vi "BMU诊断标定.vi"(5 "timeout":u32, 6 "Socket":dbl, 7 "通用配置?":bool, 8 "CAN端口":u16(ring), 9 "设备索引号":u16(ring), 10 "CAN卡类型":u32(ring)=21, 11 "从板号":u8=1) -> (3 "成功?":bool)   [LabVIEW 2013] (continued)
                    frame "从板信息" {
                    }
                    frame "电压个数" {
                    }
                    frame "通道电压节数" {
                    }
                    frame "保险位置" {
                    }
                    frame "温度个数" {
                    }
                    frame "风机关闭温差", "风机关闭温度", "风机开启温差", "风机开启温度", "加热关闭温差", "加热关闭温度", "加热开启温度", "加热控制参数" {
                    }
                    frame "SOC过低", "电压不均衡", "电压过低", "电压过高", "温度不均衡", "温度过低", "温度过高", "一级故障阀值" {
                    }
                    frame "SOC过低(2)", "电压不均衡(2)", "电压过低(2)", "电压过高(2)", "二级故障阀值", "温度不均衡(2)", "温度过低(2)", "温度过高(2)" {
                    }
                    frame "SOC过低(3)", "电压不均衡(3)", "电压过低(3)", "电压过高(3)", "三级故障阀值", "温度不均衡(3)", "温度过低(3)", "温度过高(3)" {
                    }
                    frame "快换参数" {
                    }
                    frame "均衡参数" {
                    }
                    frame "充电结束电压" {
                    }
                    frame "均衡阀值" {
                    }
                    frame "电池包信息1" {
                    }
                    frame "电池包序号" {
                    }
                    frame "充放电安时" {
                    }
                    frame "充电次数时间" {
                    }
                    frame "SOC" {
                    }
                    frame "车牌号" {
                    }
                    frame "充电参数" {
                    }
                  }
                  n3542 = local read "从板号"() -> (w4999:u8)
                }
              }
              n3543 = Build Array(w4914) -> (w4913:i32[])
              n3544 = local write "命令"(w4916) -> ()
              n3545 = Array Size(array=w4911) -> (size(s)=w4910:i32)
              n3546 = for {
                tunnel: w4911 -> [w5075] mode=indexing
                tunnel: w4916 -> [w5074]
                tunnel: w4915 -> [w5073]
                tunnel: w4913 -> [w5072]
                tunnel: w4912 -> [w5071] mode=indexing
                tunnel: w4910 -> [w5070]
                tunnel: w4909 -> [w5068]
                tunnel: [w5067] -> w4908
                i -> [w5069]
                n3547 = while {
                  tunnel: w5075 -> [w5084]
                  tunnel: w5074 -> [w5083]
                  tunnel: w5073 -> [w5082]
                  tunnel: w5072 -> [w5081]
                  tunnel: w5071 -> [w5080]
                  tunnel: w5070 -> [w5079]
                  tunnel: w5069 -> [w5078]
                  tunnel: w5068 -> [w5077]
                  tunnel: [w5076] -> w5067
                  stop <- w5076 stop-if-true
                  n3548 = stacked-sequence {
                    seq-local: [_ _ _ _ w5232 _ _] -> [_ _ _ _ _ w5241 _]
                    tunnel: w5084 -> [_ _ _ w5220 _ _ _]
                    tunnel: w5083 -> [_ _ _ w5219 _ _ _]
                    tunnel: w5082 -> [_ _ _ w5218 _ _ _]
                    tunnel: w5081 -> [_ _ _ w5217 _ _ _]
                    tunnel: [_ _ _ _ w5233 _ _] -> w5076
                    tunnel: w5080 -> [w5086 _ _ _ _ w5242 _]
                    tunnel: w5079 -> [_ _ _ _ _ _ w5252]
                    tunnel: w5078 -> [_ _ _ _ _ _ w5251]
                    tunnel: w5077 -> [w5085 _ _ _ _ _ _]
                    frame #0 {
                      n3549 = case shown="\"主板\", 默认" w5085 {
                        tunnel: w5086 -> [w5087 w5178]
                        frame "主板", Default {
                          n3550 = case shown="\"电压个数\"" w5087 {
                            frame "假", Default {
                            }
                            frame "产品编号" {
                              n3551 = control-ref of="产品编号"() -> (w5089:refnum<vi>)
                              n3552 = property class="Str"(reference=w5089, "Value"="") -> ()  [unwired: 1 in, 2 out]
                            }
                            frame "电压个数" {
                              n3553 = local read "从板个数"() -> (w5090:dbl)
                              n3554 = control-ref of="项目信息"() -> (w5094:refnum<vi>)
                              n3555 = for {
                                N: w5090 -> [_]
                                tunnel: [""] -> w5093 mode=indexing
                              }
                              n3556 = call "表格数据输入-8.6.vi"("行数"=u32 0, "列数"=u32 1, "字符串数组"=w5093, "表格引用"=w5094) -> ()  [unwired: 8 in]
                            }
                            frame "通道电压数" {
                              n3557 = control-ref of="项目信息"() -> (w5100:refnum<vi>)
                              n3558 = for {
                                N: 20 -> [_]
                                tunnel: [""] -> w5099 mode=indexing
                              }
                              n3559 = local read "从板个数"() -> (w5101:dbl)
                              n3560 = Increment(x=w5101) -> (x+1=w5097:dbl)
                              n3561 = call "表格数据输入-8.6.vi"("行数"=w5097, "列数"=u32 1, "字符串数组"=w5099, "表格引用"=w5100) -> ()  [unwired: 8 in]
                            }
                            frame "电压起始值" {
                              n3562 = local read "从板个数"() -> (w5105:dbl)
                              n3563 = Increment(x=w5105) -> (x+1=w5104:dbl)
                              n3564 = control-ref of="项目信息"() -> (w5111:refnum<vi>)
                              n3565 = for {
                                N: w5104 -> [_]
                                tunnel: [""] -> w5110 mode=indexing
                              }
                              n3566 = Multiply(x=u8 1, y=w5105) -> (x*y=w5107:dbl)
                              n3567 = Add(x=w5107, y=u8 21) -> (x+y=w5103:dbl)
                              n3568 = call "表格数据输入-8.6.vi"("行数"=w5103, "列数"=u32 1, "字符串数组"=w5110, "表格引用"=w5111) -> ()  [unwired: 8 in]
                            }
                            frame "温度个数" {
                              n3569 = local read "从板个数"() -> (w5115:dbl)
                              n3570 = Increment(x=w5115) -> (x+1=w5114:dbl)
                              n3571 = control-ref of="项目信息"() -> (w5121:refnum<vi>)
                              n3572 = for {
                                N: w5114 -> [_]
                                tunnel: [""] -> w5120 mode=indexing
                              }
                              n3573 = Multiply(x=u8 2, y=w5115) -> (x*y=w5117:dbl)
                              n3574 = Add(x=w5117, y=u8 22) -> (x+y=w5113:dbl)
                              n3575 = call "表格数据输入-8.6.vi"("行数"=w5113, "列数"=u32 1, "字符串数组"=w5120, "表格引用"=w5121) -> ()  [unwired: 8 in]
                            }
                            frame "温度起始值" {
                              n3576 = local read "从板个数"() -> (w5125:dbl)
                              n3577 = Increment(x=w5125) -> (x+1=w5124:dbl)
                              n3578 = control-ref of="项目信息"() -> (w5131:refnum<vi>)
                              n3579 = for {
                                N: w5124 -> [_]
                                tunnel: [""] -> w5130 mode=indexing
                              }
                              n3580 = Multiply(x=u8 3, y=w5125) -> (x*y=w5127:dbl)
                              n3581 = Add(x=w5127, y=u8 23) -> (x+y=w5123:dbl)
                              n3582 = call "表格数据输入-8.6.vi"("行数"=w5123, "列数"=u32 1, "字符串数组"=w5130, "表格引用"=w5131) -> ()  [unwired: 8 in]
                            }
                            frame "保险位置" {
                              n3583 = local read "从板个数"() -> (w5135:dbl)
                              n3584 = control-ref of="项目信息"() -> (w5141:refnum<vi>)
                              n3585 = for {
                                N: 10 -> [_]
                                tunnel: [""] -> w5140 mode=indexing
                              }
                              n3586 = Multiply(x=u8 4, y=w5135) -> (x*y=w5137:dbl)
                              n3587 = Add(x=w5137, y=u8 24) -> (x+y=w5134:dbl)
                              n3588 = call "表格数据输入-8.6.vi"("行数"=w5134, "列数"=u32 1, "字符串数组"=w5140, "表格引用"=w5141) -> ()  [unwired: 8 in]
                            }
                            frame "电池额定实际容量" {
                              w5143 = 0.0 ("值")
                              n3589 = control-ref of="电池实际容量(A)"() -> (w5144:refnum<vi>)
                              n3590 = control-ref of="电池额定容量(A)"() -> (w5145:refnum<vi>)
                              n3591 = property class="DigNum (严格)"(reference=w5144, "Value"=w5143) -> ()  [unwired: 1 in, 2 out]
                              n3592 = property class="DigNum (严格)"(reference=w5145, "Value"=w5143) -> ()  [unwired: 1 in, 2 out]
                            }
                            frame "SOC" {
                              n3593 = control-ref of="SOC(%)"() -> (w5146:refnum<vi>)
                              n3594 = property class="DigNum (严格)"(reference=w5146, "Value"=0.0 ("值")) -> ()  [unwired: 1 in, 2 out]
                            }
                            frame "配置文件版本" {
                              n3595 = control-ref of="配置文件版本"() -> (w5148:refnum<vi>)
                              n3596 = property class="Str"(reference=w5148, "Value"="" ("值")) -> ()  [unwired: 1 in, 2 out]
                            }
                            frame "参数修改记录" {
                              n3597 = control-ref of="使用者"() -> (w5151:refnum<vi>)
                              n3598 = control-ref of="系统时钟"() -> (w5152:refnum<vi>)
                              n3599 = property class="DigNum (严格)"(reference=w5151, "Value"=0.0 ("值")) -> ()  [unwired: 1 in, 2 out]
                              n3600 = property class="Str"(reference=w5152, "Value"="" ("值")) -> ()  [unwired: 1 in, 2 out]
                            }
                            frame "校正时钟" {
                              n3601 = control-ref of="系统时钟"() -> (w5154:refnum<vi>)
                              n3602 = property class="Str"(reference=w5154, "Value"="" ("值")) -> ()  [unwired: 1 in, 2 out]
                            }
                            frame "车牌号" {
                              n3603 = control-ref of="车架(牌)号"() -> (w5156:refnum<vi>)
                              n3604 = property class="Str"(reference=w5156, "Value"="" ("值")) -> ()  [unwired: 1 in, 2 out]
                            }
                            frame "SOH" {
                              n3605 = control-ref of="SOH(%)"() -> (w5159:refnum<vi>)
                              n3606 = property class="DigNum (严格)"(reference=w5159, "Value"=0.0 ("值")) -> ()  [unwired: 1 in, 2 out]
                            }
                            frame "一级故障阀值" {
                              n3607 = local write "一级故障"(T10 {"总电压过高"=0.0, "整组电压不均衡"=0.0, "SOC过高"=0.0, "单体电压过高"=0.0, "总电压过低"=0.0, "温度过高"=0.0, "温度过低"=0.0, "单组电压不均衡"=0.0, "整组温度不均衡"=0.0, "单组温度不均衡"=0.0, "单体电压过低"=0.0, "充电电流过高"=0.0, "放电电流过高"=0.0, "SOC过低"=0.0, "内阻过大"=0.0, "极柱温度过高"=0.0, "SOH过低"=0.0} ("一级故障")) -> ()
                            }
                            frame "二级故障阀值" {
                              n3608 = local write "一级故障 2"(T10 {"总电压过高"=0.0, "整组电压不均衡"=0.0, "SOC过高"=0.0, "单体电压过高"=0.0, "总电压过低"=0.0, "温度过高"=0.0, "温度过低"=0.0, "单组电压不均衡"=0.0, "整组温度不均衡"=0.0, "单组温度不均衡"=0.0, "单体电压过低"=0.0, "充电电流过高"=0.0, "放电电流过高"=0.0, "SOC过低"=0.0, "内阻过大"=0.0, "极柱温度过高"=0.0, "SOH过低"=0.0} ("一级故障")) -> ()
                            }
                            frame "三级故障阀值" {
                              n3609 = local write "一级故障 3"(T10 {"总电压过高"=0.0, "整组电压不均衡"=0.0, "SOC过高"=0.0, "单体电压过高"=0.0, "总电压过低"=0.0, "温度过高"=0.0, "温度过低"=0.0, "单组电压不均衡"=0.0, "整组温度不均衡"=0.0, "单组温度不均衡"=0.0, "单体电压过低"=0.0, "充电电流过高"=0.0, "放电电流过高"=0.0, "SOC过低"=0.0, "内阻过大"=0.0, "极柱温度过高"=0.0, "SOH过低"=0.0} ("一级故障")) -> ()
                            }
                            frame "加热控制参数" {
                              n3610 = local write "加热控制参数"(T11 {"风机开启温度"=0.0, "风机关闭温度"=0.0, "加热开启温度"=0.0, "加热关闭温度"=0.0, "风机开启温差"=0.0, "风机关闭温差"=0.0, "加热关闭温差"=0.0} ("加热控制参数")) -> ()
                            }
                            frame "充电控制参数" {
                              n3611 = local write "一级故障 5"(T12 {"最大允许单体电压"=0.0, "最大允许总电压"=0.0, "最小允许单体电压"=0.0, "最大允许充电电流"=0.0, "最小允许充电电流"=0.0, "最大允许充电温度"=0.0, "最小允许充电温度"=0.0, "电流步长"=0.0} ("一级故障 5")) -> ()
                            }
                            frame "电池信息1" {
                              w5165 = ""
                              w5166 = 0.0 ("电池串联")
                              n3612 = local read "电池信息"() -> (w5168:T13)
                              n3613 = Bundle By Name(cluster=w5168, "电池串联"=w5166, "电池并联"=w5166, "电池包额定容量"=w5166, "电池包额定能量(kWh)"=w5166, "电池包额定总电压"=w5166, "实际容量"=w5166, "电池厂家"=w5165, "电池类型"=w5165, "电池生产日期"=w5165) -> (w5167:T13)
                              n3614 = local write "电池信息"(w5167) -> ()
                            }
                            frame "电池包组号" {
                              n3615 = local read "电池信息"() -> (w5171:T13)
                              n3616 = Bundle By Name(cluster=w5171, "电池包组号"="") -> (w5170:T13)
                              n3617 = local write "电池信息"(w5170) -> ()
                            }
                            frame "充放电安时" {
                              w5172 = 0.0 ("累计充电总安时")
                              n3618 = local read "电池信息"() -> (w5174:T13)
                              n3619 = Bundle By Name(cluster=w5174, "累计充电总安时"=w5172, "累计放电总安时"=w5172) -> (w5173:T13)
                              n3620 = local write "电池信息"(w5173) -> ()
                            }
                            frame "电池充放电次数" {
                              w5175 = 0.0 ("累计充电总安时")
                              n3621 = local read "电池信息"() -> (w5177:T13)
                              n3622 = Bundle By Name(cluster=w5177, "电池充满次数"=w5175, "电池放空次数"=w5175, "电池充电次数"=w5175) -> (w5176:T13)
                              n3623 = local write "电池信息"(w5176) -> ()
                            }
                          }
                        }
                        frame "从板" {
                          n3624 = case shown="\"加热控制参数\"" w5178 {
                            frame "假", Default {
                            }
                            frame "电压起始值" {
                              n3625 = control-ref of="项目信息 2"() -> (w5180:refnum<vi>)
                              n3626 = for {
                                N: 1 -> [_]
                                tunnel: [""] -> w5183 mode=indexing
                              }
                              n3627 = call "表格数据输入-8.6.vi"("行数"=u32 0, "列数"=u32 1, "字符串数组"=w5183, "表格引用"=w5180) -> ()  [unwired: 8 in]
                            }
                            frame "通道电压节数" {
                              n3628 = control-ref of="项目信息 2"() -> (w5185:refnum<vi>)
                              n3629 = for {
                                N: 5 -> [_]
                                tunnel: [""] -> w5189 mode=indexing
                              }
                              n3630 = call "表格数据输入-8.6.vi"("行数"=u32 22, "列数"=u32 1, "字符串数组"=w5189, "表格引用"=w5185) -> ()  [unwired: 8 in]
                            }
                            frame "保险位置" {
                              n3631 = control-ref of="项目信息 2"() -> (w5191:refnum<vi>)
                              n3632 = for {
                                N: 20 -> [_]
                                tunnel: [""] -> w5195 mode=indexing
                              }
                              n3633 = call "表格数据输入-8.6.vi"("行数"=u32 2, "列数"=u32 1, "字符串数组"=w5195, "表格引用"=w5191) -> ()  [unwired: 8 in]
                            }
                            frame "温度起始值" {
                              n3634 = control-ref of="项目信息 2"() -> (w5197:refnum<vi>)
                              n3635 = for {
                                N: 1 -> [_]
                                tunnel: [""] -> w5201 mode=indexing
                              }
                              n3636 = call "表格数据输入-8.6.vi"("行数"=u32 1, "列数"=u32 1, "字符串数组"=w5201, "表格引用"=w5197) -> ()  [unwired: 8 in]
                            }
                            frame "加热控制参数" {
                              n3637 = local write "加热控制参数"(T11 {"风机开启温度"=0.0, "风机关闭温度"=0.0, "加热开启温度"=0.0, "加热关闭温度"=0.0, "风机开启温差"=0.0, "风机关闭温差"=0.0, "加热关闭温差"=0.0} ("加热控制参数")) -> ()
                            }
                            frame "一级故障阀值" {
                              n3638 = local write "一级故障 6"(T15 {"电压过高"=0.0, "电压过低"=0.0, "温度过高"=0.0, "温度过低"=0.0, "电压不均衡(V)"=0.0, "温度不均衡"=0.0, "SOC过低"=0.0} ("一级故障 6")) -> ()
                            }
                            frame "二级故障阀值" {
                              n3639 = local write "一级故障 7"(T15 {"电压过高"=0.0, "电压过低"=0.0, "温度过高"=0.0, "温度过低"=0.0, "电压不均衡(V)"=0.0, "温度不均衡"=0.0, "SOC过低"=0.0} ("一级故障 7")) -> ()
                            }
                            frame "三级故障阀值" {
                              n3640 = local write "一级故障 8"(T15 {"电压过高"=0.0, "电压过低"=0.0, "温度过高"=0.0, "温度过低"=0.0, "电压不均衡(V)"=0.0, "温度不均衡"=0.0, "SOC过低"=0.0} ("一级故障 7")) -> ()
                            }
                            frame "均衡参数" {
                              n3641 = local write "均衡参数"(T17 {"充电结束电压(90%)"=0.0, "充电结束电压(91%)"=0.0, "充电结束电压(92%)"=0.0, "充电结束电压(93%)"=0.0, "充电结束电压(94%)"=0.0, "均衡计算-电压高阀值1级"=0.0, "均衡计算-电压高阀值2级"=0.0, "均衡计算-电压低阀值1级"=0.0, "均衡计算-电压低阀值2级"=0.0, "均衡计算-最低电压阀值"=0.0, "均衡停止-最低电压阀值"=0.0, "均衡计算-电压极差阀值"=0.0, "充电结束电压(95%)"=0.0, "充电结束电压(96%)"=0.0, "充电结束电压(97%)"=0.0, "充电结束电压(98%)"=0.0, "充电结束电压(99%)"=0.0, "充电结束电压(100%)"=0.0} ("均衡参数")) -> ()
                            }
                            frame "均衡阀值" {
                              w5208 = sgl 0.0 ("均衡计算-电压高阀值1级")
                              n3642 = local read "均衡参数"() -> (w5209:T17)
                              n3643 = Bundle By Name(cluster=w5209, "均衡计算-电压高阀值1级"=w5208, "均衡计算-电压高阀值2级"=w5208, "均衡计算-电压低阀值1级"=w5208, "均衡计算-电压低阀值2级"=w5208, "均衡计算-最低电压阀值"=w5208, "均衡停止-最低电压阀值"=w5208, "均衡计算-电压极差阀值"=w5208) -> (w5210:T17)
                              n3644 = local write "均衡参数"(w5210) -> ()
                            }
                            frame "充电结束电压" {
                              w5211 = sgl 0.0 ("均衡计算-电压高阀值1级")
                              n3645 = local read "均衡参数"() -> (w5212:T17)
                              n3646 = Bundle By Name(cluster=w5212, "充电结束电压(90%)"=w5211, "充电结束电压(91%)"=w5211, "充电结束电压(92%)"=w5211, "充电结束电压(93%)"=w5211, "充电结束电压(94%)"=w5211, "充电结束电压(95%)"=w5211, "充电结束电压(96%)"=w5211, "充电结束电压(97%)"=w5211, "充电结束电压(98%)"=w5211, "充电结束电压(99%)"=w5211, "充电结束电压(100%)"=w5211) -> (w5213:T17)
                              n3647 = local write "均衡参数"(w5213) -> ()
                            }
                          }
                        }
                      }
                    }
                    frame #1 {
                      w5214 = FALSE ("流控帧")
                      w5215 = TRUE ("流控帧 2")
                      n3648 = global write "EV05全局变量1.vi" "写入超时"(w5214) -> ()
                      n3649 = global write "EV05全局变量1.vi" "流控帧"(w5214) -> ()
                      n3650 = local write "写?"(w5214) -> ()
                      n3651 = call <vilib>:"Set Busy.vi"("disable click? (T)"=w5214) -> ()  [unwired: 3 in, 8 out]
                      n3652 = local write "消除"(w5215) -> ()
                      n3653 = local write "控制1"(w5215) -> ()
                      n3654 = global write "EV05全局变量1.vi" "流控帧 2"(w5215) -> ()
                    }
                    frame #2 {
                      n3655 = Wait Until Next ms Multiple(millisecond multiple=u32 150 ("毫秒倍数")) -> ()  [unwired: 1 out]
                    }
                    frame #3 {
                      n3656 = local read "设备索引号"() -> (w5222:u16)
                      n3657 = local read "CAN卡类型"() -> (w5223:u32)
                      n3658 = local read "CAN端口"() -> (w5221:u16)
                      n3659 = stacked-sequence {
                        tunnel: w5223 -> [_ w5231]
                        tunnel: w5222 -> [_ w5230]
                        tunnel: w5221 -> [_ w5229]
                        tunnel: w5220 -> [_ w5228]
                        tunnel: w5219 -> [_ w5227]
                        tunnel: w5218 -> [_ w5226]
                        tunnel: w5217 -> [_ w5225]
                        frame #0 {
                        }
                        frame #1 {
                          n3660 = call "多帧发送机制(EV05).vi"("can卡类型"=w5231, "设备索引号"=w5230, "CAN端口"=w5229, "命令"=w5227, "板号"=w5226, "命令序号"=w5228, "输入数据"=w5225) -> ("错误输出"=w5224:errorcluster)  [unwired: 2 in, 10 out]
                          n3661 = call <vilib>:"Clear Errors.vi"("error in (no error)"=w5224) -> ()  [unwired: 6 in, 1 out]
                        }
                      }
                      "命令序号" <- w5220
                    }
                    frame #4 {
                      n3662 = while {
                        tunnel: [w5236] -> w5233
                        tunnel: [w5235] -> w5232
                        i -> [w5239]
                        stop <- w5236 stop-if-true
                        n3663 = local read "强制终止读写标记"() -> (w5234:bool)
                        n3664 = global read "EV05全局变量1.vi" "写入超时"() -> (w5235:bool)
                        n3665 = Greater Or Equal?(x=w5239, y=30) -> (x >= y?=w5237:bool)
                        n3666 = Compound Arithmetic op=OR(w5234, w5235, w5237) -> (w5236:bool)
                        n3667 = Wait Until Next ms Multiple(millisecond multiple=u32 100 ("毫秒倍数")) -> ()  [unwired: 1 out]
                      }
                    }
                    frame #5 {
                      n3668 = call <vilib>:"Unset Busy.vi"() -> ()  [unwired: 11 in, 1 out]
                      n3669 = case shown="假" w5241 {
                        tunnel: w5242 -> [w5245 _]
                        frame False {
                          n3670 = control-ref of="结果"() -> (w5244:refnum<vi>)
                          n3671 = Concatenate Strings(w5245, "     读取失败" ("字符串")) -> (w5247:string)
                          n3672 = Build Array(w5247) -> (w5243:string[])
                          n3673 = call "表格编辑.vi"("新元素/子数组"=w5243, "活动单元格:单元格背景色"=u32 16740749, "MCListbox引用句柄"=w5244) -> ()  [unwired: 9 out]
                        }
                        frame True {
                        }
                      }
                    }
                    frame #6 {
                      n3674 = Increment(x=w5251) -> (x+1=w5250:i32)
                      n3675 = Equal?(x=w5252, y=w5250) -> (x = y?=w5249:bool)
                      n3676 = case shown="真" w5249 {
                        frame False {
                        }
                        frame True {
                          n3677 = control-ref of="结果"() -> (w5254:refnum<vi>)
                          n3678 = Concatenate Strings("读取完成" ("字符串")) -> (w5256:string)
                          n3679 = Build Array(w5256) -> (w5253:string[])
                          n3680 = call "表格编辑.vi"("新元素/子数组"=w5253, "活动单元格:单元格背景色"=u32 21937, "MCListbox引用句柄"=w5254) -> ()  [unwired: 9 out]
                        }
                      }
                    }
                  }
                }
              }
            }
          }
          n3681 = stacked-sequence {
            tunnel: w4906 -> [_]
            frame #0 {
              n3682 = call <vilib>:"Unset Busy.vi"() -> ()  [unwired: 11 in, 1 out]
              n3683 = local write "强制终止读写标记"(FALSE ("强制停止")) -> ()
            }
          }
        }
        frame "全部读取" {
          n3684 = stacked-sequence {
            seq-local: [w5262 _ _] -> [_ _ w5817]
            seq-local: [w5261 _ _] -> [_ _ w5816]
            tunnel: [_ w5453 _] -> w5259
            frame #0 {
              n3685 = local read "主从选择"() -> (w5262:enum32{"主板", "从板"})
              n3686 = local read "路径"() -> (w5263:path)
              n3687 = Empty String/Path?(string/path=w5263) -> (empty?=w5261:bool)
              n3688 = disable-structure shown="禁用" {
                disable-tunnel: w5263 -> [w5266 _]
                disable-tunnel: w5261 -> [w5265 _]
                disable-tunnel: w5262 -> [w5264 _]
                frame Disabled {
                  n3689 = case shown="假" w5265 {
                    tunnel: w5266 -> [w5270 _]
                    tunnel: w5264 -> [w5269 _]
                    frame False {
                      n3690 = control-ref of="结果"() -> (w5267:refnum<vi>)
                      n3691 = call-poly <vilib>:"Read From Spreadsheet File.vi"("file path (dialog if empty)"=w5270) -> ("all rows"=w5268:string[][])  [unwired: 3 in, 7 out]
                      n3692 = case shown="\"主板\", 默认" w5269 {
                        tunnel: w5268 -> [w5272 w5367]
                        tunnel: w5267 -> [w5271 w5366]
                        frame "主板", Default {
                          n3693 = stacked-sequence {
                            tunnel: w5272 -> [w5281 w5305 w5362]
                            tunnel: w5271 -> [w5278 _ w5333]
                            frame #0 {
                              n3694 = Index Array(array=w5281, index (col)=3 ("禁用的索引 (列)")) -> (element=w5295:string[])  [unwired: 1 in]
                              n3695 = Index Array(array=w5281, index (col)=1 ("禁用的索引 (列)")) -> (element=w5301:string[])  [unwired: 1 in]
                              n3696 = Delete From Array(array=w5295, length=4 ("长度"), index=0 ("索引")) -> (deleted portion=w5292:string[], array with subset deleted=w5286:string[])
                              n3697 = Delete From Array(array=w5301, length=1 ("长度"), index=0 ("索引")) -> (deleted portion=w5298:string[], array with subset deleted=w5275:string[])
                              n3698 = Build Array("正在读取主板配置文件...") -> (w5279:string[])
                              n3699 = Index Array(array=w5286) -> (element #1=w5285:string, element #2=w5284:string, element #3=w5283:string, element #4=w5282:string)  [unwired: 4 in]
                              n3700 = for {
                                tunnel: w5292 -> [w5304] mode=indexing
                                tunnel: [w5303] -> w5291 mode=indexing
                                n3701 = Fract/Exp String To Number(string=w5304) -> (number=w5303:dbl)  [unwired: 4 out]
                              }
                              n3702 = Index Array(array=w5298) -> (element=w5297:string)  [unwired: 1 in]
                              n3703 = global write "读配置文件全局.vi" "表格输入"(w5275) -> ()
                              n3704 = call "表格编辑.vi"("新元素/子数组"=w5279, "活动单元格:单元格背景色"=u32 6618880, "MCListbox引用句柄"=w5278) -> ()  [unwired: 9 out]
                              n3705 = Decimal String To Number(string=w5297) -> (number=w5276:i32)  [unwired: 1 in, 2 out]
                              n3706 = global read "读配置文件全局.vi" "项目信息"() -> (w5274:T27)
                              n3707 = Index Array(array=w5291) -> (element #1=w5290:dbl, element #2=w5289:dbl, element #3=w5288:dbl, element #4=w5287:dbl)  [unwired: 4 in]
                              n3708 = global write "读配置文件全局.vi" "从板个数"(w5276) -> ()
                              n3709 = Bundle(cluster=w5274, "电池额定容量"=w5290, "电池实际容量"=w5289, "车牌号"=w5285, "配置文件版本"=w5284, "SOH"=w5287, "SOC"=w5288, "产品编号"=w5283, "系统时钟"=w5282) -> (w5273:T27)  [unwired: 1 out]
                              n3710 = global write "读配置文件全局.vi" "项目信息"(w5273) -> ()
                            }
                            frame #1 {
                              n3711 = Index Array(array=w5305, index (col)=3 ("禁用的索引 (列)")) -> (element=w5323:string[])  [unwired: 1 in]
                              n3712 = Index Array(array=w5305, index (col)=5 ("禁用的索引 (列)")) -> (element=w5317:string[])  [unwired: 1 in]
                              n3713 = for {
                                tunnel: w5317 -> [w5330] mode=indexing
                                tunnel: [w5329] -> w5316 mode=indexing
                                n3714 = Fract/Exp String To Number(string=w5330) -> (number=w5329:dbl)  [unwired: 4 out]
                              }
                              n3715 = Delete From Array(array=w5323, length=17 ("长度"), index=8 ("索引")) -> (deleted portion=w5321:string[])  [unwired: 1 out]
                              n3716 = for {
                                tunnel: w5321 -> [w5332] mode=indexing
                                tunnel: [w5331] -> w5319 mode=indexing
                                n3717 = Fract/Exp String To Number(string=w5332) -> (number=w5331:dbl)  [unwired: 4 out]
                              }
                              n3718 = global write "读配置文件全局.vi" "二级故障"(w5316) -> ()
                              n3719 = global write "读配置文件全局.vi" "一级故障"(w5319) -> ()
                              n3720 = Index Array(array=w5305, index (col)=7 ("禁用的索引 (列)")) -> (element=w5314:string[])  [unwired: 1 in]
                              n3721 = Index Array(array=w5305, index (col)=9 ("禁用的索引 (列)")) -> (element=w5311:string[])  [unwired: 1 in]
                              n3722 = for {
                                tunnel: w5314 -> [w5328] mode=indexing
                                tunnel: [w5327] -> w5313 mode=indexing
                                n3723 = Fract/Exp String To Number(string=w5328) -> (number=w5327:dbl)  [unwired: 4 out]
                              }
                              n3724 = for {
                                tunnel: w5311 -> [w5326] mode=indexing
                                tunnel: [w5325] -> w5310 mode=indexing
                                n3725 = Fract/Exp String To Number(string=w5326) -> (number=w5325:dbl)  [unwired: 4 out]
                              }
                              n3726 = Delete From Array(array=w5310, length=6 ("长度"), index=0 ("索引")) -> (deleted portion=w5307:dbl[], array with subset deleted=w5306:dbl[])
                              n3727 = global write "读配置文件全局.vi" "三级故障"(w5313) -> ()
                              n3728 = global write "读配置文件全局.vi" "加热控制参数"(w5307) -> ()
                              n3729 = global write "读配置文件全局.vi" "充电控制参数"(w5306) -> ()
                            }
                            frame #2 {
                              n3730 = call <vilib>:"Unset Busy.vi"() -> ()  [unwired: 2 in, 10 out]
                              n3731 = Index Array(array=w5362, index (col)=11 ("禁用的索引 (列)")) -> (element=w5359:string[])  [unwired: 1 in]
                              n3732 = Delete From Array(array=w5359, length=6 ("长度"), index=0 ("索引")) -> (deleted portion=w5341:string[], array with subset deleted=w5340:string[])
                              n3733 = for {
                                tunnel: w5340 -> [w5365] mode=indexing
                                tunnel: [w5364] -> w5358 mode=indexing
                                n3734 = Fract/Exp String To Number(string=w5365) -> (number=w5364:dbl)  [unwired: 4 out]
                              }
                              n3735 = Index Array(array=w5341) -> (element #1=w5357:string, element #2=w5356:string, element #3=w5355:string, element #4=w5354:string, element #5=w5353:string, element #6=w5352:string)  [unwired: 6 in]
                              n3736 = Index Array(array=w5358) -> (element #1=w5351:dbl, element #2=w5350:dbl, element #3=w5349:dbl, element #4=w5348:dbl, element #5=w5347:dbl, element #6=w5346:dbl, element #7=w5345:dbl, element #8=w5344:dbl, element #9=w5343:dbl, element #10=w5342:dbl, element #11=w5337:dbl)  [unwired: 11 in]
                              n3737 = global read "读配置文件全局.vi" "电池信息"() -> (w5339:T28)
                              n3738 = Build Array("配置文件读取完成") -> (w5335:string[])
                              n3739 = Bundle(cluster=w5339, "电池串联"=w5351, "电池并联"=w5350, "累计放电总安时"=w5348, "电池包额定容量"=w5347, "电池包额定能量"=w5346, "电池包额定总电压"=w5345, "累计充电总安时"=w5349, "电池充满次数"=w5344, "电池放空次数"=w5343, "电池充电次数"=w5342, "电池生产日期"=w5357, "电池厂家"=w5356, "电池类型"=w5355, "电池包组号"=w5354, "电池包产权标识"=w5353, "电池应用车型"=w5352, "实际容量"=w5337) -> (w5338:T28)
                              n3740 = call "表格编辑.vi"("新元素/子数组"=w5335, "活动单元格:单元格背景色"=u32 6618880, "MCListbox引用句柄"=w5333) -> ()  [unwired: 9 out]
                              n3741 = global write "读配置文件全局.vi" "电池信息"(w5338) -> ()
                            }
                          }
                        }
                        frame "从板" {
                          n3742 = stacked-sequence {
                            tunnel: w5367 -> [w5375 w5403 w5447]
                            tunnel: w5366 -> [w5372 _ w5423]
                            frame #0 {
                              n3743 = Index Array(array=w5375, index (col)=1 ("禁用的索引 (列)")) -> (element=w5385:string[])  [unwired: 1 in]
                              n3744 = Index Array(array=w5375, index (col)=3 ("禁用的索引 (列)")) -> (element=w5379:string[])  [unwired: 1 in]
                              n3745 = Delete From Array(array=w5385, length=1 ("长度"), index=0 ("索引")) -> (deleted portion=w5382:string[], array with subset deleted=w5369:string[])
                              n3746 = Delete From Array(array=w5379, length=6 ("长度"), index=0 ("索引")) -> (deleted portion=w5376:string[])  [unwired: 1 out]
                              n3747 = for {
                                tunnel: w5376 -> [w5388] mode=indexing
                                tunnel: [w5387] -> w5368 mode=indexing
                                i -> [w5389]
                                n3748 = Fract/Exp String To Number(string=w5388, default (0 dbl)=w5389) -> (number=w5387:i32)  [unwired: 3 out]
                              }
                              n3749 = Index Array(array=w5382) -> (element=w5381:string)  [unwired: 1 in]
                              n3750 = global write "读配置文件全局2.vi" "表格"(w5369) -> ()
                              n3751 = Build Array("正在读取从板配置文件...") -> (w5373:string[])
                              n3752 = Decimal String To Number(string=w5381) -> (number=w5370:i32)  [unwired: 1 in, 2 out]
                              n3753 = call "表格编辑.vi"("新元素/子数组"=w5373, "活动单元格:单元格背景色"=u32 6618880, "MCListbox引用句柄"=w5372) -> ()  [unwired: 9 out]
                              n3754 = global write "读配置文件全局2.vi" "加热控制参数"(w5368) -> ()
                              n3755 = global write "读配置文件全局2.vi" "从板板号"(w5370) -> ()
                            }
                            frame #1 {
                              n3756 = Index Array(array=w5403, index (col)=3 ("禁用的索引 (列)")) -> (element=w5393:string[])  [unwired: 1 in]
                              n3757 = Array Subset(array=w5393, index=6 ("索引"), length=7 ("长度")) -> (w5400:string[])
                              n3758 = Array Subset(array=w5393, index=13 ("索引"), length=7 ("长度")) -> (w5399:string[])
                              n3759 = Array Subset(array=w5393, index=20 ("索引"), length=7 ("长度")) -> (w5394:string[])
                              n3760 = for {
                                tunnel: w5400 -> [w5410] mode=indexing
                                tunnel: [w5409] -> w5390 mode=indexing
                                n3761 = Fract/Exp String To Number(string=w5410) -> (number=w5409:dbl)  [unwired: 4 out]
                              }
                              n3762 = for {
                                tunnel: w5399 -> [w5408] mode=indexing
                                tunnel: [w5407] -> w5391 mode=indexing
                                n3763 = Fract/Exp String To Number(string=w5408) -> (number=w5407:dbl)  [unwired: 4 out]
                              }
                              n3764 = for {
                                tunnel: w5394 -> [w5406] mode=indexing
                                tunnel: [w5405] -> w5392 mode=indexing
                                n3765 = Fract/Exp String To Number(string=w5406) -> (number=w5405:dbl)  [unwired: 4 out]
                              }
                              n3766 = global write "读配置文件全局2.vi" "一级故障阀值"(w5390) -> ()
                              n3767 = global write "读配置文件全局2.vi" "二级故障阀值"(w5391) -> ()
                              n3768 = global write "读配置文件全局2.vi" "三级故障阀值"(w5392) -> ()
                            }
                            frame #2 {
                              n3769 = Index Array(array=w5447, index (col)=5 ("禁用的索引 (列)")) -> (element=w5445:string[])  [unwired: 1 in]
                              n3770 = Delete From Array(array=w5445, length=1 ("长度"), index=16 ("索引")) -> (deleted portion=w5441:string[], array with subset deleted=w5442:string[])
                              n3771 = for {
                                tunnel: w5442 -> [w5450] mode=indexing
                                tunnel: [w5449] -> w5446 mode=indexing
                                n3772 = Fract/Exp String To Number(string=w5450) -> (number=w5449:dbl)  [unwired: 4 out]
                              }
                              n3773 = Index Array(array=w5446) -> (element #1=w5440:dbl, element #2=w5439:dbl, element #3=w5438:dbl, element #4=w5437:dbl, element #5=w5436:dbl, element #6=w5435:dbl, element #7=w5434:dbl, element #8=w5433:dbl, element #9=w5432:dbl, element #10=w5431:dbl, element #11=w5430:dbl, element #12=w5421:dbl, element #13=w5429:dbl, element #14=w5428:dbl, element #15=w5427:dbl, element #16=w5426:dbl, element #17=w5419:dbl, element #18=w5418:dbl, element #19=w5417:dbl, element #20=w5416:dbl, element #21=w5415:dbl, element #22=w5414:dbl)  [unwired: 22 in]
                              n3774 = Build Array("配置文件读取完成") -> (w5424:string[])
                              n3775 = Index Array(array=w5441, index=22 ("索引")) -> (element=w5420:string)
                              n3776 = global read "读配置文件全局2.vi" "电池组信息"() -> (w5412:T29)
                              n3777 = call "表格编辑.vi"("新元素/子数组"=w5424, "活动单元格:单元格背景色"=u32 6618880, "MCListbox引用句柄"=w5423) -> ()  [unwired: 9 out]
                              n3778 = Bundle(cluster=w5412, "电池类型"=w5440, "电池厂家"=w5439, "电池地区"=w5438, "电池组序号"=w5437, "电池包串联数"=w5436, "电池包并联数"=w5435, "电池包安时数"=w5434, "电池包序号"=w5433, "充电次数"=w5432, "充满电时间"=w5431, "放空时间"=w5430, "车牌号"=w5420, "最大允许单体电压"=w5421, "最大允许总电压"=w5429, "最大允许温度"=w5428, "最小允许温度"=w5427, "最大允许充电电流"=w5426, "最小允许充电电流"=w5419, "最小允许单体电压"=w5418, "电流步长"=w5417, "SOC"=w5416, "充电总安时"=w5415, "放电总这时"=w5414) -> (w5411:T29)
                              n3779 = call <vilib>:"Unset Busy.vi"() -> ()  [unwired: 2 in, 10 out]
                              n3780 = global write "读配置文件全局2.vi" "电池组信息"(w5411) -> ()
                            }
                          }
                        }
                      }
                    }
                    frame True {
                    }
                  }
                }
                frame Enabled {
                }
              }
              n3781 = case shown="\"从板\"" w5262 {
                frame "主板", Default {
                  w5451 = FALSE
                  n3782 = global write "读配置文件全局.vi" "SOC判定"(w5451) -> ()
                  n3783 = global write "读配置文件全局.vi" "SOH判定"(w5451) -> ()
                  n3784 = global write "读配置文件全局.vi" "车牌号判定"(w5451) -> ()
                  n3785 = global write "读配置文件全局.vi" "电池信息1判定"(w5451) -> ()
                  n3786 = global write "读配置文件全局.vi" "保险位置判定"(w5451) -> ()
                  n3787 = global write "读配置文件全局.vi" "产品编号判定"(w5451) -> ()
                  n3788 = global write "读配置文件全局.vi" "充放电安时判定"(w5451) -> ()
                  n3789 = global write "读配置文件全局.vi" "从板个数判定"(w5451) -> ()
                  n3790 = global write "读配置文件全局.vi" "电池包组号判定"(w5451) -> ()
                  n3791 = global write "读配置文件全局.vi" "电压个数判定"(w5451) -> ()
                  n3792 = global write "读配置文件全局.vi" "电压起始值判定"(w5451) -> ()
                  n3793 = global write "读配置文件全局.vi" "二级故障判定"(w5451) -> ()
                  n3794 = global write "读配置文件全局.vi" "三级故障判定"(w5451) -> ()
                  n3795 = global write "读配置文件全局.vi" "通道电压数判定"(w5451) -> ()
                  n3796 = global write "读配置文件全局.vi" "温度个数判定"(w5451) -> ()
                  n3797 = global write "读配置文件全局.vi" "一级故障判定"(w5451) -> ()
                  n3798 = global write "读配置文件全局.vi" "温度起始值判定"(w5451) -> ()
                  n3799 = global write "读配置文件全局.vi" "充电控制参数判定"(w5451) -> ()
                  n3800 = global write "读配置文件全局.vi" "电池充放电次数判定"(w5451) -> ()
                  n3801 = global write "读配置文件全局.vi" "加热控制参数判定"(w5451) -> ()
                  n3802 = global write "读配置文件全局.vi" "配置文件版本判定"(w5451) -> ()
                  n3803 = global write "读配置文件全局.vi" "电池额定实际容量判定"(w5451) -> ()
                }
                frame "从板" {
                  w5452 = FALSE
                  n3804 = disable-structure shown="禁用" {
                    frame Disabled {
                      n3805 = global read "读配置文件全局2.vi" "充电次数时间判定"() -> ()  [unwired: 1 in]
                      n3806 = global read "读配置文件全局2.vi" "电池包信息1判定"() -> ()  [unwired: 1 in]
                      n3807 = global read "读配置文件全局2.vi" "电池包序号判定"() -> ()  [unwired: 1 in]
                      n3808 = global read "读配置文件全局2.vi" "充放电安时判定"() -> ()  [unwired: 1 in]
                      n3809 = global read "读配置文件全局2.vi" "车牌号判定"() -> ()  [unwired: 1 in]
                      n3810 = global read "读配置文件全局2.vi" "充电参数判定"() -> ()  [unwired: 1 in]
                      n3811 = global read "读配置文件全局2.vi" "保险位置判定"() -> ()  [unwired: 1 in]
                    }
                    frame Enabled {
                    }
                  }
                  n3812 = global write "读配置文件全局2.vi" "从板号判定"(w5452) -> ()
                  n3813 = global write "读配置文件全局2.vi" "通道电压判定"(w5452) -> ()
                  n3814 = global write "读配置文件全局2.vi" "保险位置判定"(w5452) -> ()
                  n3815 = global write "读配置文件全局2.vi" "二级故障判定"(w5452) -> ()
                  n3816 = global write "读配置文件全局2.vi" "三级故障判定"(w5452) -> ()
                  n3817 = global write "读配置文件全局2.vi" "一级故障判定"(w5452) -> ()
                  n3818 = global write "读配置文件全局2.vi" "电压起始值判定"(w5452) -> ()
                  n3819 = global write "读配置文件全局2.vi" "温度起始值判定"(w5452) -> ()
                }
              }
            }
            frame #1 {
              (unwired) "均衡参数"
              # "去掉加热控制信息 20140106"
              n3820 = local read "主从选择"() -> (w5456:enum32{"主板", "从板"})
              n3821 = case shown="\"主板\", 默认" w5456 {
                tunnel: [string[] ["项目信息", "一级故障阀值", "二级故障阀值", "三级故障阀值", "加热控制信息", "充电控制信息", "电池信息"] string[] ["从板信息", "一级故障阀值", "二级故障阀值", "三级故障阀值"]] -> w5455
                frame "主板", Default {
                }
                frame "从板" {
                }
              }
              n3822 = Array Size(array=w5455) -> (size(s)=w5454:i32)
              n3823 = for {
                tunnel: w5455 -> [w5472] mode=indexing
                tunnel: w5456 -> [w5460]
                tunnel: w5454 -> [w5464]
                tunnel: [w5459] -> w5453
                i -> [w5461]
                n3824 = case shown="\"主板\", 默认" w5460 {
                  tunnel: [w5768 w5796] -> w5466
                  tunnel: [w5767 w5797] -> w5467
                  tunnel: w5472 -> [w5764 w5793]
                  tunnel: [u8 0 ("板号") w5794] -> w5471
                  tunnel: [u8 0 ("板号") u8 0 ("板号")] -> w5470
                  tunnel: [w5763 w5792] -> w5468
                  frame "主板", Default {
                    n3825 = case shown="\"项目信息\"" w5764 {
                      tunnel: [_ u8[] [1, 2, 3, 4, 5, 6, 13, 8, 7, 9, 10, 11, 12] u8[] [1] u8[] [2] u8[] [3] u8[] [1] u8[] [2] u8[] [1, 2, 3] u8[] [1, 2, 3, 4]] -> w5768
                      tunnel: [_ u8 128 ("命令") u8 129 ("命令") u8 129 ("命令") u8 129 ("命令") u8 130 ("命令") u8 130 ("命令") u8 131 ("命令") u8 132 ("命令")] -> w5767
                      tunnel: [_ string[] ["产品编号", "电压个数", "通道电压数", "电压起始值", "温度个数", "温度起始值", "保险位置", "电池额定实际容量", "SOC", "配置文件版本", "参数修改记录", "车牌号", "SOH"] string[] ["一级故障阀值"] string[] ["二级故障阀值"] string[] ["三级故障阀值"] string[] ["加热控制参数"] string[] ["充电控制参数"] _ string[] ["电池信息1", "电池包组号", "充放电安时", "电池充放电次数"]] -> w5763
                      frame "假", Default {
                      }
                      frame "项目信息" {
                      }
                      frame "一级故障阀值" {
                      }
                      frame "二级故障阀值" {
                      }
                      frame "三级故障阀值" {
                      }
                      frame "加热控制信息" {
                      }
                      frame "充电控制信息" {
                      }
                      frame "历史信息" {
                      }
                      frame "电池信息" {
                      }
                    }
                  }
                  frame "从板" {
                    n3826 = case shown="\"从板信息\"" w5793 {
                      tunnel: [_ u8 0 ("命令") u8 2 ("命令") u8 2 ("命令") u8 2 ("命令") u8 3 ("命令") u8 6 ("命令")] -> w5797
                      tunnel: [_ u8[] [6, 1, 2, 3, 4, 5] u8[] [1] u8[] [2] u8[] [3] u8[] [1, 2, 3, 4, 5, 6, 7] u8[] [1, 2]] -> w5796
                      tunnel: [_ string[] ["从板号", "电压起始值", "通道电压节数", "保险位置", "温度起始值", "加热控制参数"] string[] ["一级故障阀值"] string[] ["二级故障阀值"] string[] ["三级故障阀值"] string[] ["电池包信息1", "电池包序号", "充放电安时", "充电次数时间", "SOC", "车牌号", "充电参数"] string[] ["均衡阀值", "充电结束电压"]] -> w5792
                      frame "假", Default {
                      }
                      frame "从板信息" {
                      }
                      frame "一级故障阀值" {
                      }
                      frame "二级故障阀值" {
                      }
                      frame "三级故障阀值" {
                      }
                      frame "快换参数" {
                      }
                      frame "均衡参数" {
                      }
                    }
                    n3827 = local read "从板号"() -> (w5794:u8)
                  }
                }
                n3828 = Increment(x=w5461) -> (x+1=w5463:i32)
                n3829 = Equal?(x=w5464, y=w5463) -> (x = y?=w5462:bool)
                n3830 = case shown="\"从板\"" w5460 {
                  tunnel: w5461 -> [w5734 w5748]
                  frame "主板", Default {
                    n3831 = case shown="0, 默认" w5734 {
                      tunnel: [T8."项目信息" ("主从板") T8."一级故障阀值" ("主从板") T8."二级故障阀值" ("主从板") T8."三级故障阀值" ("主从板") T8."控制参数" ("主从板") T8."电池信息" ("主从板")] -> w5733
                      frame 0, Default {
                        n3832 = local write "1"(TRUE ("1")) -> ()
                      }
                      frame 1 {
                        n3833 = local write "1 2"(TRUE ("1 2")) -> ()
                      }
                      frame 2 {
                        n3834 = local write "1 3"(TRUE ("1 3")) -> ()
                      }
                      frame 3 {
                        n3835 = local write "1 4"(TRUE ("1 4")) -> ()
                      }
                      frame 4, 5 {
                        n3836 = local write "1 5"(TRUE ("1 5")) -> ()
                      }
                      frame 6 {
                        n3837 = local write "1 11"(TRUE ("1 11")) -> ()
                      }
                    }
                    n3838 = local write "主板2"(w5733) -> ()
                  }
                  frame "从板" {
                    n3839 = case shown="4" w5748 {
                      tunnel: [T21."从板信息" ("等级 2") T21."从板信息" ("等级 2") T21."一级故障阀值" ("等级 2") T21."二级故障阀值" ("等级 2") T21."三级故障阀值" ("等级 2") T21."快换参数" ("等级 2") T14."均衡参数" ("等级 2")] -> w5747
                      frame 99, Default {
                        n3840 = local write "1 6"(TRUE ("1 6")) -> ()
                      }
                      frame 0 {
                        n3841 = local write "1 6"(TRUE ("1 6")) -> ()
                      }
                      frame 1 {
                        n3842 = local write "1 7"(TRUE ("1 7")) -> ()
                      }
                      frame 2 {
                        n3843 = local write "1 8"(TRUE ("1 8")) -> ()
                      }
                      frame 3 {
                        n3844 = local write "1 9"(TRUE ("1 9")) -> ()
                      }
                      frame 5 {
                        n3845 = local write "1 10"(TRUE ("1 10")) -> ()
                      }
                      frame 4 {
                        n3846 = local write "1 12"(TRUE ("1 10")) -> ()
                      }
                    }
                    n3847 = local write "等级 2"(w5747) -> ()
                  }
                }
                n3848 = Array Size(array=w5466) -> (size(s)=w5465:i32)
                n3849 = local write "命令"(w5467) -> ()
                n3850 = Build Array(w5470) -> (w5469:u8[])
                n3851 = while {
                  tunnel: w5467 -> [w5504]
                  tunnel: w5471 -> [w5503]
                  tunnel: w5469 -> [w5502]
                  tunnel: w5465 -> [w5498]
                  tunnel: w5462 -> [w5501]
                  tunnel: w5460 -> [w5495]
                  tunnel: [w5494] -> w5459
                  shift-right: [w5493] -> _
                  shift-left: w5468 -> [w5474]
                  shift-right: [w5484] -> _
                  shift-left: w5466 -> [w5473]
                  i -> [w5499]
                  stop <- w5494 stop-if-true
                  n3852 = local read "强制终止读写标记"() -> (w5490:bool)
                  n3853 = Array Size(array=w5474) -> (size(s)=w5492:i32)
                  n3854 = Increment(x=w5499) -> (x+1=w5500:i32)
                  n3855 = Greater Than 0?(x=w5492) -> (x > 0?=w5491:bool)
                  n3856 = Equal?(x=w5498, y=w5500) -> (x = y?=w5496:bool)
                  n3857 = Not(x=w5490) -> (.not. x?=w5489:bool)
                  n3858 = And(x=w5489, y=w5491) -> (x .and. y?=w5488:bool)
                  n3859 = Delete From Array(array=w5474, length=1 ("长度"), index=0 ("索引")) -> (deleted portion=w5480:string[], array with subset deleted=w5485:string[])
                  n3860 = Index Array(array=w5480, index=0 ("索引")) -> (element=w5478:string)
                  n3861 = Delete From Array(array=w5473, length=1 ("长度"), index=0 ("索引")) -> (deleted portion=w5476:u8[], array with subset deleted=w5481:u8[])
                  n3862 = Index Array(array=w5476, index=0 ("索引")) -> (element=w5475:u8)
                  n3863 = case shown="真" w5488 {
                    tunnel: w5504 -> [_ w5520]
                    tunnel: w5475 -> [_ w5519]
                    tunnel: w5503 -> [_ w5518]
                    tunnel: w5502 -> [_ w5517]
                    tunnel: w5478 -> [_ w5516]
                    tunnel: w5501 -> [_ w5515]
                    tunnel: w5496 -> [_ w5514]
                    tunnel: w5495 -> [_ w5513]
                    tunnel: [string[] [] w5509] -> w5493
                    tunnel: w5485 -> [_ w5512]
                    tunnel: [u8[] [] w5507] -> w5484
                    tunnel: w5481 -> [_ w5511]
                    tunnel: w5474 -> [_ w5510]
                    tunnel: w5473 -> [_ w5508]
                    frame False {
                    }
                    frame True {
                      n3864 = while {
                        tunnel: w5520 -> [w5536]
                        tunnel: w5519 -> [w5535]
                        tunnel: w5518 -> [w5534]
                        tunnel: w5517 -> [w5533]
                        tunnel: w5516 -> [w5531]
                        tunnel: w5515 -> [w5530]
                        tunnel: w5514 -> [w5529]
                        tunnel: w5513 -> [w5528]
                        tunnel: w5512 -> [w5524]
                        tunnel: w5511 -> [w5522]
                        tunnel: w5510 -> [w5525]
                        tunnel: [w5526] -> w5509
                        tunnel: w5508 -> [w5523]
                        tunnel: [w5521] -> w5507
                        i -> [w5527]
                        stop <- w5532 stop-if-true
                        n3865 = stacked-sequence {
                          seq-local: [_ _ _ _ w5683 _ _] -> [_ _ _ _ _ w5699 _]
                          tunnel: w5536 -> [_ _ _ w5675 _ _ _]
                          tunnel: w5535 -> [_ _ _ w5674 _ _ _]
                          tunnel: w5534 -> [_ _ _ w5673 _ _ _]
                          tunnel: w5533 -> [_ _ _ w5672 _ _ _]
                          tunnel: [_ _ _ _ w5684 _ _] -> w5532
                          tunnel: w5531 -> [w5538 _ _ _ _ w5698 _]
                          tunnel: w5530 -> [_ _ _ _ _ _ w5726]
                          tunnel: w5529 -> [_ _ _ _ _ _ w5724]
                          tunnel: w5528 -> [w5537 _ _ _ _ _ _]
                          tunnel: w5527 -> [_ _ _ _ _ _ _]
                          tunnel: [_ _ _ _ _ w5697 _] -> w5526
                          tunnel: w5525 -> [_ _ _ _ _ w5696 _]
                          tunnel: w5524 -> [_ _ _ _ _ w5695 _]
                          tunnel: w5523 -> [_ _ _ _ _ w5694 _]
                          tunnel: w5522 -> [_ _ _ _ _ w5693 _]
                          tunnel: [_ _ _ _ _ w5692 _] -> w5521
                          frame #0 {
                            n3866 = case shown="\"主板\", 默认" w5537 {
                              tunnel: w5538 -> [w5539 w5630]
                              frame "主板", Default {
                                n3867 = case shown="\"电池包组号\"" w5539 {
                                frame "假", Default {
                                }
                                frame "产品编号" {
                                n3868 = control-ref of="产品编号"() -> (w5541:refnum<vi>)
                                n3869 = property class="Str"(reference=w5541, "Value"="") -> ()  [unwired: 1 in, 2 out]
                                }
                                frame "电压个数" {
                                n3870 = local read "从板个数"() -> (w5542:dbl)
                                n3871 = control-ref of="项目信息"() -> (w5546:refnum<vi>)
                                n3872 = for {
                                N: w5542 -> [_]
                                tunnel: [""] -> w5545 mode=indexing
                                }
                                n3873 = call "表格数据输入-8.6.vi"("行数"=u32 0, "列数"=u32 1, "字符串数组"=w5545, "表格引用"=w5546) -> ()  [unwired: 8 in]
                                }
                                frame "通道电压数" {
                                n3874 = disable-structure shown="禁用" {
                                frame Disabled {
                                n3875 = control-ref of="项目信息"() -> (w5552:refnum<vi>)
                                n3876 = for {
                                N: 20 -> [_]
                                tunnel: [""] -> w5551 mode=indexing
                                }
                                n3877 = local read "从板个数"() -> (w5553:dbl)
                                n3878 = Increment(x=w5553) -> (x+1=w5549:dbl)
                                n3879 = call "表格数据输入-8.6.vi"("行数"=w5549, "列数"=u32 1, "字符串数组"=w5551, "表格引用"=w5552) -> ()  [unwired: 8 in]
                                }
                                frame Enabled {
                                }
                                }
                                }
